vi "Dispose Module Images.vi"(5 "Archive":bool, 7 "Dispose":bool, 8 "error in":errorcluster, 11 "Potting Procedure in":refnum<class "Potting Procedure.lvclass">) -> (0 "error out":errorcluster, 3 "Potting Procedure out":refnum<class "Potting Procedure.lvclass">)   [LabVIEW 2011, in "Potting Procedure.lvclass"]
uses:
  Potting Procedure.lvclass
  Shared Components/Gantry Class/Gantry Class.lvclass
  Shared Components/Vec3d Class/Vec3d Class.lvclass
  Shared Components/Config Manager Class/Config Manager Class.lvclass
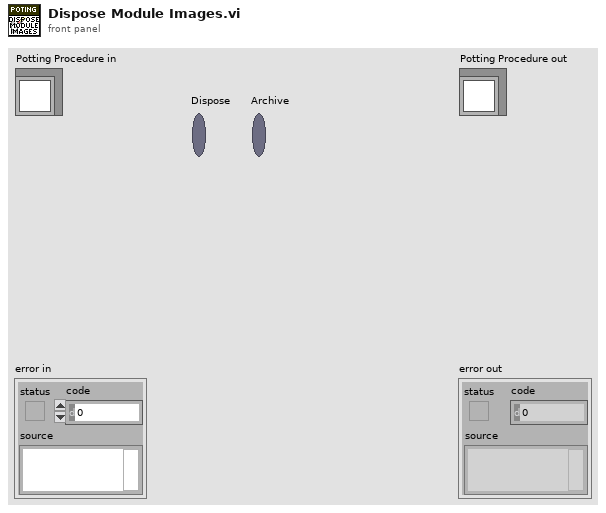
[diagram p1: front panel]
types:
  T1 = typedef "Inspect Modules.ctl" = cluster{"Has Been Run?":bool, "Module Positions":T2[]}
  T2 = typedef "Inspect Modules - Module.ctl" = cluster{"TBM-TBM":T3, "TBM-HDI":T3, "Address Pads":T3, "HDI Bond Pad References":T7[], "BBM Bond Pad References":T7[], "HV-HDI":T7, "HV-BBM":T7, "Chuck":i32, "Slot":i32, "Potting Selection":cluster{"HDI Bond Pads":bool[], "BBM Bond Pads":bool[], "TBM Inner":cluster{"Top":bool, "Left":bool, "Bottom":bool, "Right":bool}, "TBM Outer":cluster{"Top":bool, "Left":bool, "Bottom":bool, "Right":bool}, "Address Pads":cluster{"Top":bool, "Bottom":bool}, "High Voltage":cluster{"HDI":bool, "BBM":bool}}}
  T3 = typedef "Multi-Fiducial Image.ctl" = cluster{"Fiducial Image":T4, "Fiducials":cluster{"Selected Fiducial":T6, "fiducial name":string}[]}
  T4 = typedef "Physical Image.ctl" = cluster{"Image Position":refnum<class "Vec3d Class.lvclass">, "Image Reference":T5, "Field of View":cluster{"x(mm)":dbl, "y(mm)":dbl}}
  T5 = typedef "IMAQ Image.ctl" = refnum<image>
  T6 = typedef "Fiducial with Source.ctl" = cluster{"Fiducial Image Coordinate":refnum<class "Vec3d Class.lvclass">, "Fiducial Source":enum16{"Pattern Recognition", "User", "Error", "Default"}}
  T7 = typedef "Fiducial Image.ctl" = cluster{"Fiducial Image":T4, "Selected Fiducial":T6, "fiducial name":string}
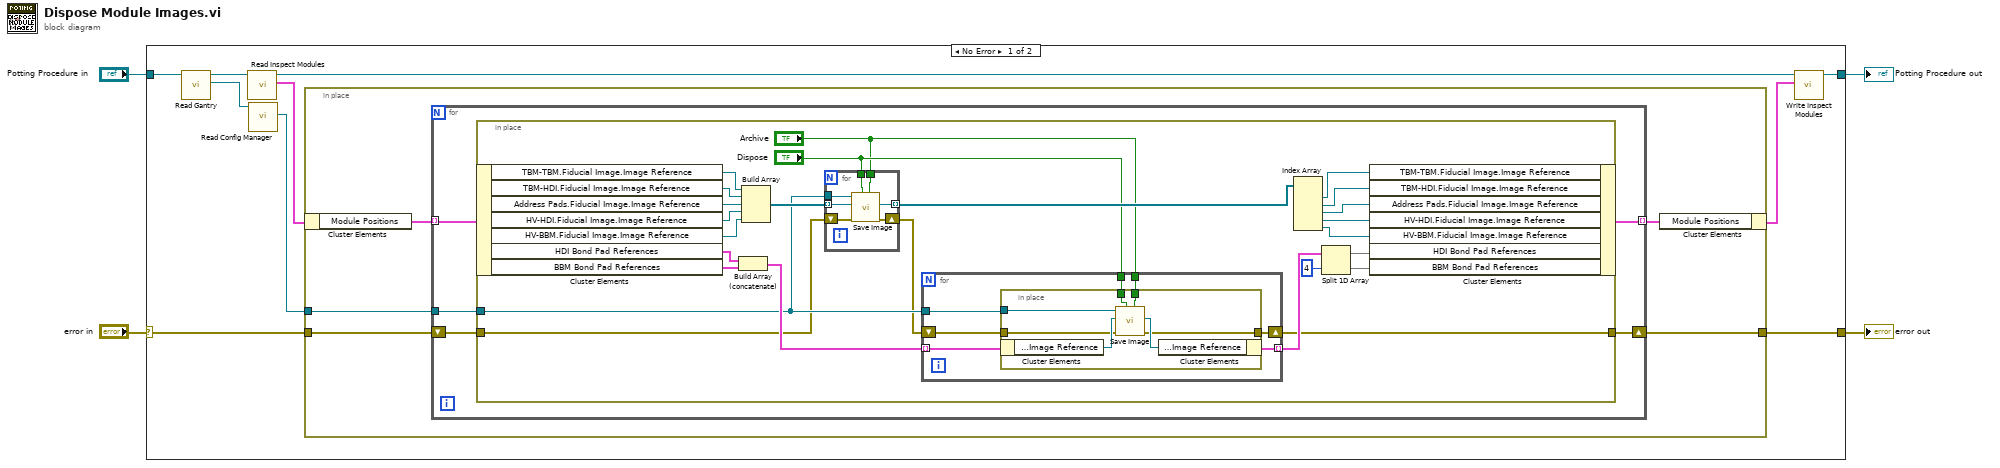
[diagram p0: block diagram]
diagram:
  n1 = case shown="No Error" "error in" {
    selector: "error in" -> [w10 w72]
    tunnel: [w9 w72] -> w3
    tunnel: [w11 w71] -> w1
    tunnel: "Potting Procedure in" -> [w8 w71]
    frame No Error {
      n2 = call-dynamic "Read Gantry.vi"("Potting Procedure in"=w8) -> ("Gantry"=w6:refnum<class "Gantry Class.lvclass">, "Potting Procedure out"=w7:refnum<class "Potting Procedure.lvclass">)  [unwired: 8 in, 1 out]
      n3 = call-dynamic "Read Inspect Modules.vi"("Potting Procedure in"=w7) -> ("Inspect Modules"=w14:T1, "Potting Procedure out"=w12:refnum<class "Potting Procedure.lvclass">)  [unwired: 8 in, 1 out]
      n4 = call-dynamic "Read Config Manager.vi"("Gantry in"=w6) -> ("Config Manager"=w5:refnum<class "Config Manager Class.lvclass">)  [unwired: 8 in, 2 out]
      n5 = in-place {
        in-place-border: w10 -> [w17]
        in-place-border: [w16] -> w9
        in-place-border: w5 -> [w15]
        n6 = in-place-cluster #1(w14) -> ("Module Positions"=w19:T2[])
        n7 = for {
          tunnel: w19 -> [w24] mode=indexing
          tunnel: [w23] -> w18 mode=indexing
          shift-right: [w20] -> w16
          shift-left: w17 -> [w22]
          tunnel: w15 -> [w21]
          n8 = in-place {
            in-place-border: w22 -> [w35]
            in-place-border: w21 -> [w36]
            in-place-border: [w27] -> w20
            n9 = in-place-cluster #2(w24) -> ("TBM-TBM.Fiducial Image.Image Reference"=w49:T5, "TBM-HDI.Fiducial Image.Image Reference"=w48:T5, "Address Pads.Fiducial Image.Image Reference"=w47:T5, "HV-HDI.Fiducial Image.Image Reference"=w46:T5, "HV-BBM.Fiducial Image.Image Reference"=w45:T5, "HDI Bond Pad References"=w43:T7[], "BBM Bond Pad References"=w42:T7[])
            n10 = Build Array (concatenate)(w43, w42) -> (w44:T7[])
            n11 = Build Array(w49, w48, w47, w46, w45) -> (w37:T5[])
            n12 = for {
              tunnel: w37 -> [w52] mode=indexing
              tunnel: w36 -> [w56]
              shift-right: [w54] -> w34
              shift-left: w35 -> [w55]
              tunnel: [w53] -> w33 mode=indexing
              tunnel: "Dispose" -> [w51]
              tunnel: "Archive" -> [w50]
              n13 = call "Save Image.vi"("Archive"=w50, "Dispose"=w51, "error in"=w55, "Image in"=w52, "Config Manager in"=w56) -> ("error out"=w54:errorcluster, "Image out"=w53:T5)  [unwired: 4 in, 1 out]
            }
            n14 = for {
              tunnel: w44 -> [w63] mode=indexing
              tunnel: [w62] -> w41 mode=indexing
              tunnel: w36 -> [w61]
              shift-right: [w59] -> w27
              shift-left: w34 -> [w60]
              tunnel: "Dispose" -> [w58]
              tunnel: "Archive" -> [w57]
              n15 = in-place {
                in-place-border: w61 -> [w68]
                in-place-border: w60 -> [w67]
                in-place-border: [w66] -> w59
                in-place-border: w58 -> [w65]
                in-place-border: w57 -> [w64]
                n16 = in-place-cluster #3(w63) -> ("Fiducial Image.Image Reference"=w69:T5)
                n17 = call "Save Image.vi"("Archive"=w64, "Dispose"=w65, "error in"=w67, "Image in"=w69, "Config Manager in"=w68) -> ("error out"=w66:errorcluster, "Image out"=w70:T5)  [unwired: 4 in, 1 out]
                n18 = in-place-cluster #3("Fiducial Image.Image Reference"=w70) -> (w62:T7)
              }
            }
            n19 = Index Array(array=w33) -> (element #1=w32:T5, element #2=w31:T5, element #3=w30:T5, element #4=w29:T5, element #5=w28:T5)  [unwired: 5 in]
            n20 = Split 1D Array(array=w41, index=4) -> (first subarray=w40:T7[], second subarray=w39:T7[])
            n21 = in-place-cluster #2("TBM-TBM.Fiducial Image.Image Reference"=w32, "TBM-HDI.Fiducial Image.Image Reference"=w31, "Address Pads.Fiducial Image.Image Reference"=w30, "HV-HDI.Fiducial Image.Image Reference"=w29, "HV-BBM.Fiducial Image.Image Reference"=w28, "HDI Bond Pad References"=w40, "BBM Bond Pad References"=w39) -> (w23:T2)
          }
        }
        n22 = in-place-cluster #1("Module Positions"=w18) -> (w13:T1)
      }
      n23 = call-dynamic "Write Inspect Modules.vi"("Inspect Modules"=w13, "Potting Procedure in"=w12) -> ("Potting Procedure out"=w11:refnum<class "Potting Procedure.lvclass">)  [unwired: 8 in, 1 out]
    }
    frame Error {
    }
  }
  "error out" <- w3
  "Potting Procedure out" <- w1
